vi "AttackerPenalty.vi"(4 "AI Parameters":T8={"GotoKick"={"Dist do cone a frente"=150.0, "attacker farback"=1500.0, "Perto"=300.0, "min dist to kick"=150.0, "kick eps"=0.0, "Time to transition"=0.05}, "Attacker"={"CC chute"=0.09, "CC passe"=0.045, "Kick Force"=100.0, "ball-robot Kick"=200.0, "ball-robot Pass"=0.3, "drible\nAttk"=FALSE}, "Defender"={"D max"=1700.0, "Vel p/ robô av"=1000.0, "Kick Force"=100.0, "D atk-def"=0.0, "D farback"=0.0, "drible\ndef"=FALSE, "drible\ngoalie"=FALSE}, "Timeout"={"Field/v in x"=6.0, "Dist Robots"=300, "Dist up in y"=300}, "Pose Striker"={"dist"=200.0, "Numeric"=-4.0, "dist 2"=200.0, "drible\nstriker"=FALSE}, "Dist Stop"=300.0, "D ball out"=200, "D central gap "=150.0, "T pass"=0.0, "Force ++"=0.0, "range kick"=0.0, "Chute alto"=TRUE, "Marcador novo"=TRUE, "drible"=FALSE, "D drible"=300.0, "Versão Striker"=enum."Auto", "Defesa"=enum."ManMark", "Marcador"=enum."Marcar Segundo mais perigoso", "Receptor passe"=enum."Auto", "Área"=enum."Quadrada", "Decisão\nsimples?"=FALSE} {"D drible" format="%#_13g"; "D central gap" format="%#_13g"; "Dist Stop" format="%#_13g"; "Pose Striker"."Numeric" format="%#_13g"; "Defender"."Kick Force" format="%#_13g"; "Defender"."Vel p/ robô av" format="%#_13g"; "Attacker"."ball-robot Kick" format="%#_13g"; "Attacker"."Kick Force" format="%#_13g"; "Attacker"."CC passe" format="%#_13g"; "Attacker"."CC chute" format="%#_13g"; "GotoKick"."kick eps" format="%#_13g"; "GotoKick"."min dist to kick" format="%#_13g"; "GotoKick"."Perto" format="%#_13g"; "GotoKick"."attacker farback" format="%#_13g"; "GotoKick"."Dist do cone a frente" format="%#_13g"}, 7 "IA State Input":T9={"our_robots"=[], "enemy_robots"=[], "balls"=[], "geometry"={"line_width"=0, "field_length"=0, "field_width"=0, "boundary_width"=0, "referee_width"=0, "goal_width"=0, "goal_depth"=0, "goal_wall_width"=0, "center_circle_radius"=0, "defense_radius"=0, "defense_stretch"=0, "free_kick_from_defense_dist"=0, "penalty_spot_from_field_line_dist"=0, "penalty_line_from_spot_dist"=0}, "IA Judge"={"stage"="", "command"="", "our_goalie_id"=0.0, "enemy_goalie_id"=0.0, "command enum"=enum."Halt", "Time"=enum."Azul"}, "Received Timestamp"=timestamp(0 s since 1904-01-01), "Events"={"Touch"=FALSE, "Ball out"=FALSE, "id touch"=0.0, "Ball out of \nVision"=FALSE, "Ball inside \nGoalie area"=FALSE, "Robot not responding"=FALSE, "Robots responding status"=[1.0, 1.0, 1.0, 1.0, 1.0, 1.0], "Enemy Ball \nPossession"=FALSE, "Pass State"=FALSE, "id end of pass"=0.0, "Kick"=FALSE, "Id ini Possession"=0.0, "Ball Possesion"=FALSE, "Id Possesion"=0.0, "Direct Kick"=FALSE, "2nd Strk Ativo"=FALSE}}, 8 "atacando contra?":bool=TRUE, 9 "balls":T6[](array[typedef]), 10 "geometry":T7, 11 "Robot in":T1={"id"=0, "function"=enum."Attacker", "x"=0.0, "y"=0.0, "orientation"=0.0, "v_tangent"=0.0, "v_normal"=0.0, "v_ang"=0.0, "kick_x"=0.0, "kick_z"=0.0, "dribble"=FALSE, "Timestamp"=timestamp(0 s since 1904-01-01), "estimatives"={"est_v_tangent"=0.0, "est_v_normal"=0.0, "est_vx"=0.0, "est_vy"=0.0, "Pos Robot Est"=[]}, "dest_x_kick"=0.0, "dest_y_kick"=0.0, "Gap Coord"=[], "States"=enum."GoToTangent", "Path "=[], "Path  Smooth"=[], "Dest"=[]}) -> (2 "Robot out":T1={"id"=5, "function"=enum."Attacker", "x"=-1842.5054931640625, "y"=520.60986328125, "orientation"=-2.7555055618286133, "v_tangent"=-0.08361641967936218, "v_normal"=-0.20513016702014014, "v_ang"=0.24456003022714357, "kick_x"=0.0, "kick_z"=0.0, "dribble"=FALSE, "Timestamp"=timestamp(2082758857.4639893 s since 1904-01-01), "estimatives"={"est_v_tangent"=0.0, "est_v_normal"=0.0, "est_vx"=0.0, "est_vy"=0.0, "Pos Robot Est"=[]}, "dest_x_kick"=0.0, "dest_y_kick"=0.0, "Gap Coord"=[], "States"=enum."GoToTangent", "Path "=[], "Path  Smooth"=[], "Dest"=[]})   [LabVIEW 2018]
uses:
  Core/AI Input.ctl
  Core/AI Robot.ctl
  Functions Enum.ctl
  AttackerStates.ctl
  Path Planning/RRT/PathDests.ctl
  Path Planning/RRT/PathDest.ctl
  Core/AI Ball.ctl
  Core/Field Size.ctl
  Core/AI Judge.ctl
  Command Enum.ctl
  Util/Events/Events.ctl
  AI Parameters.ctl
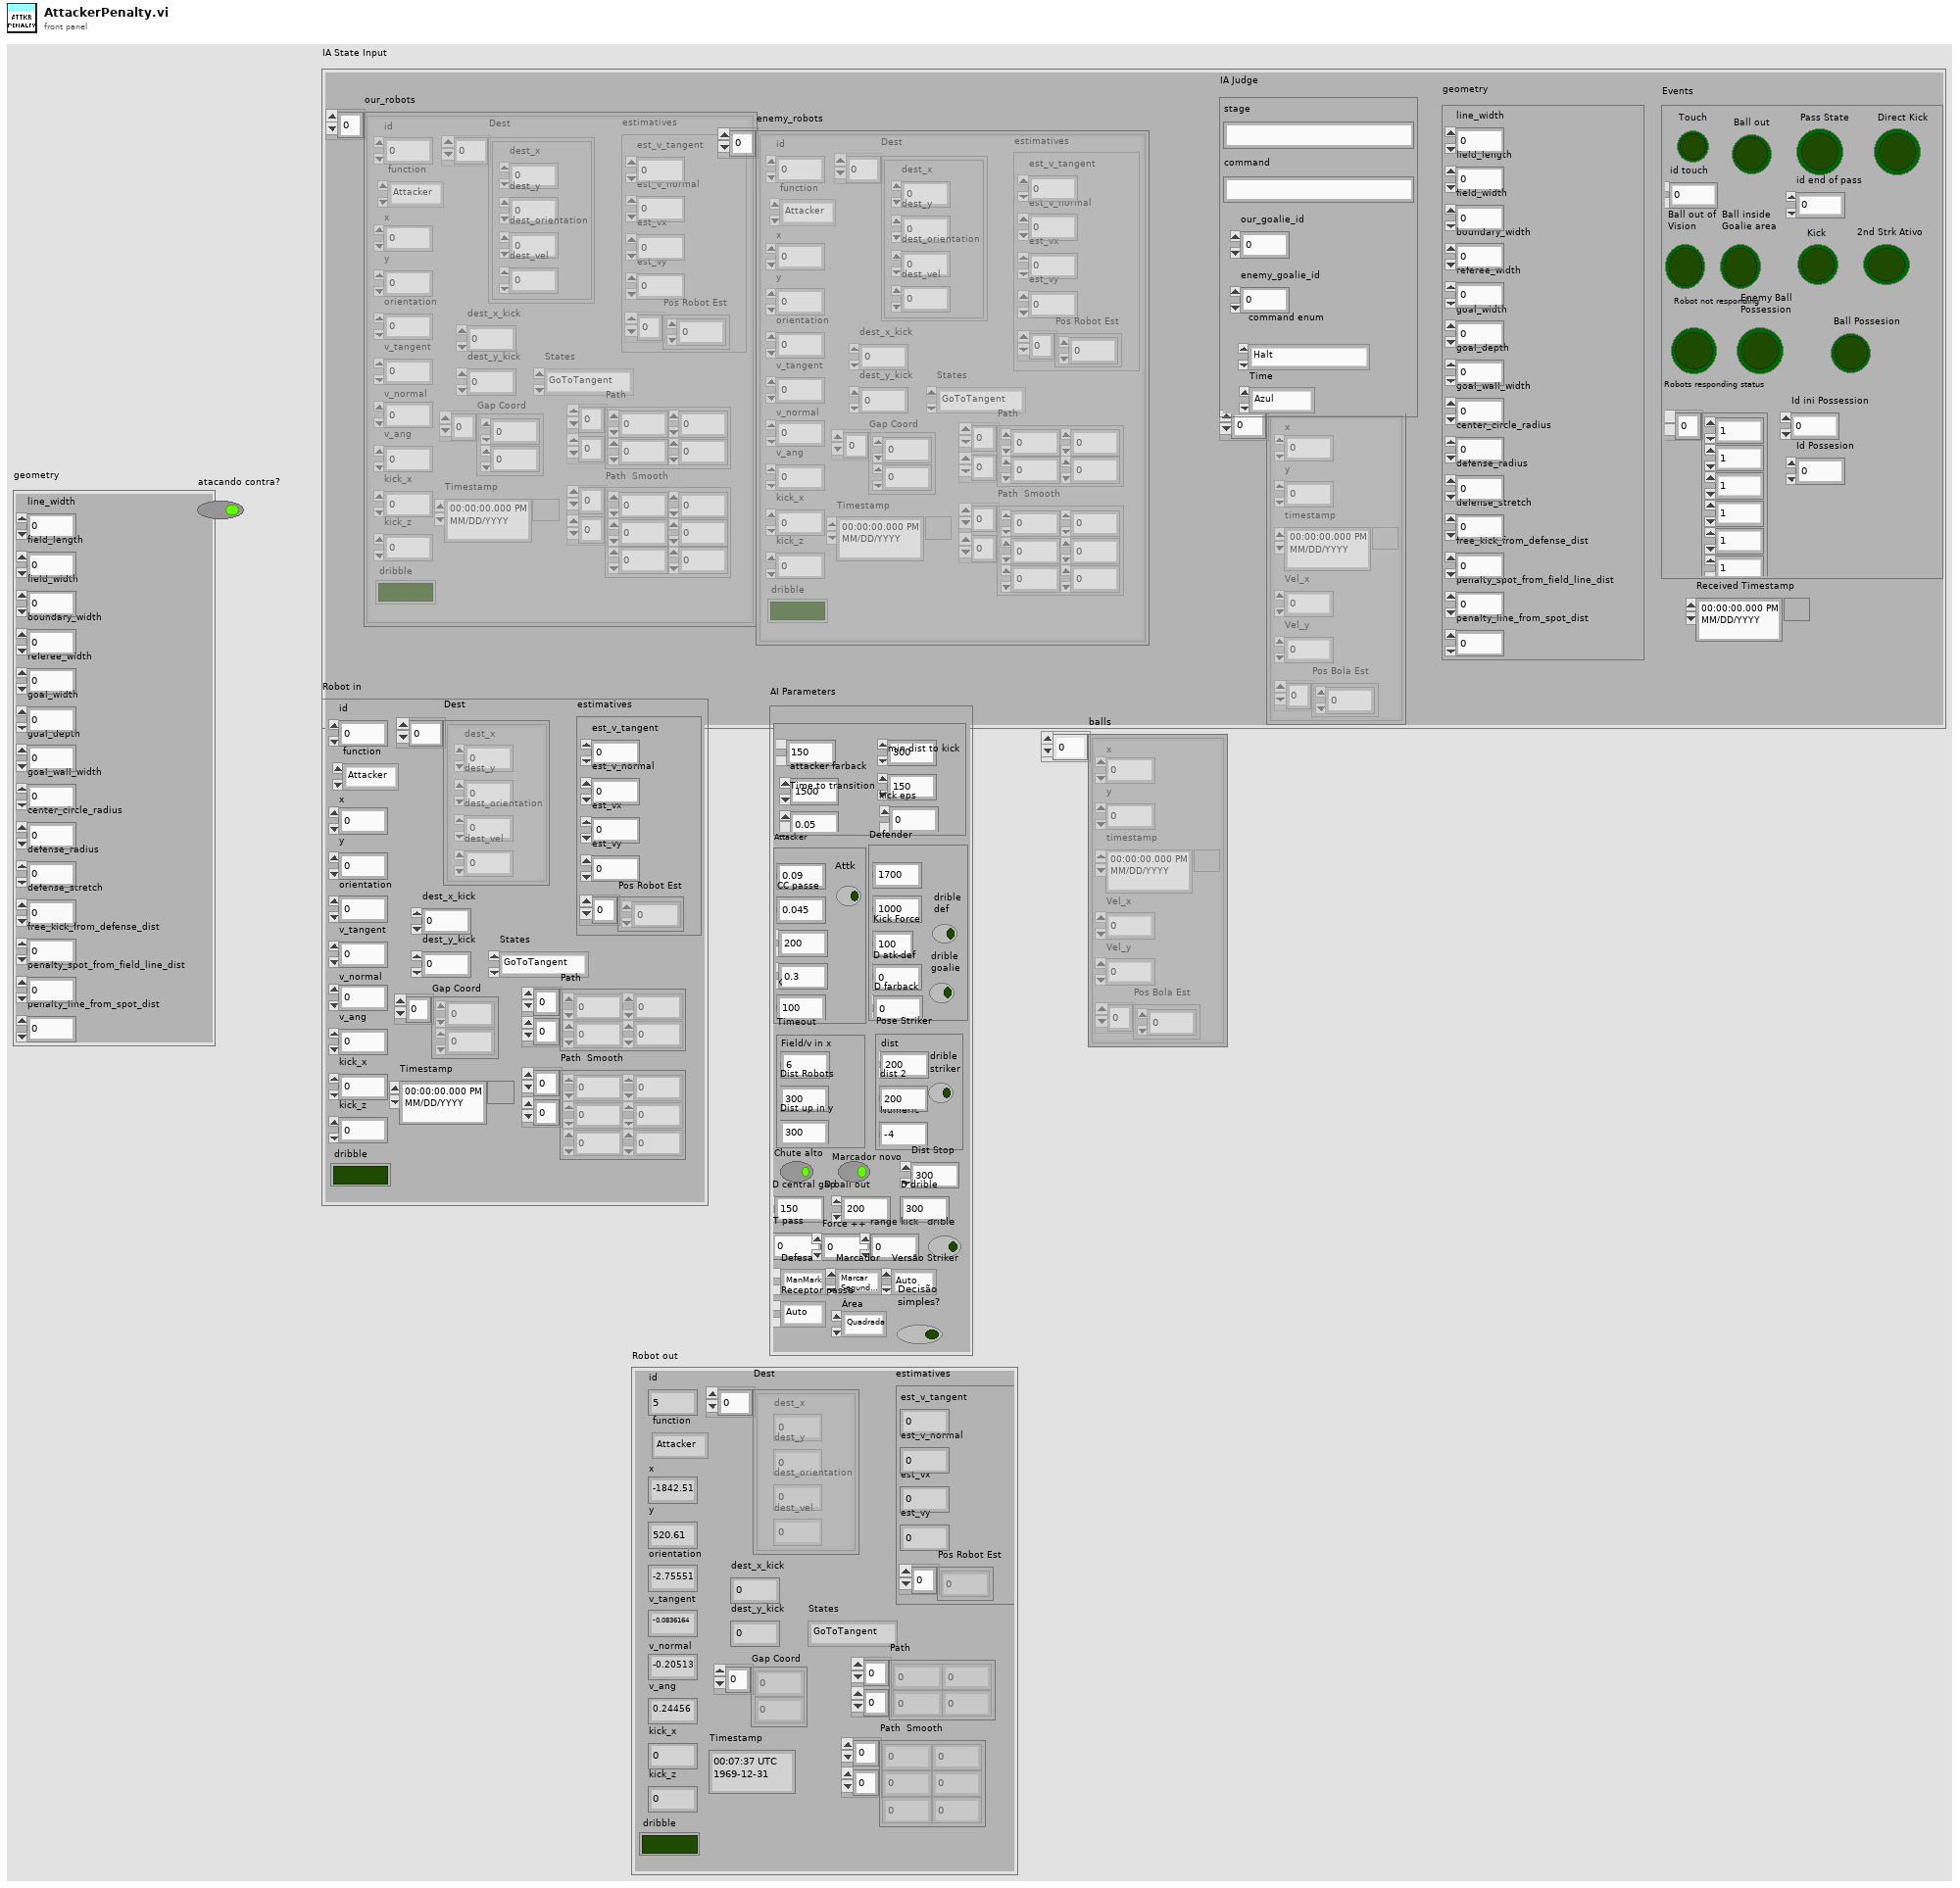
[diagram p1: front panel]
types:
  T1 = typedef "AI Robot.ctl" = cluster{"id":u32, "function":T2, "x":dbl, "y":dbl, "orientation":dbl, "v_tangent":dbl, "v_normal":dbl, "v_ang":dbl, "kick_x":dbl, "kick_z":dbl, "dribble":bool, "Timestamp":timestamp, "estimatives":cluster{"est_v_tangent":dbl, "est_v_normal":dbl, "est_vx":dbl, "est_vy":dbl, "Pos Robot Est":dbl[]}, "dest_x_kick":dbl, "dest_y_kick":dbl, "Gap Coord":dbl[], "States":T3, "Path ":dbl[][], "Path  Smooth":dbl[][], "Dest":T4}
  T2 = typedef "Functions Enum.ctl" = enum16{"2nd Striker", "Attacker", "Goalie", "Defender", "Striker", "Goto 0", "Dummy", "Kicker", "ZigZag 0", "ZigZag 1", "ZigZag 2", "ZigZag 3", "ZigZag 4", "ZigZag 5", "ZigZag 6", "ZigZag 7", "ZigZag 8", ""}
  T3 = typedef "AttackerStates.ctl" = enum16{"Pass", "GoToTangent", "BallGetting", "GoToKick", ""}
  T4 = typedef "PathDests.ctl" = T5[]
  T5 = typedef "PathDest.ctl" = cluster{"dest_x":dbl, "dest_y":dbl, "dest_orientation":dbl, "dest_vel":dbl}
  T6 = typedef "AI Ball.ctl" = cluster{"x":dbl, "y":dbl, "timestamp":timestamp, "Vel_x":dbl, "Vel_y":dbl, "Pos Bola Est":dbl[]}
  T7 = typedef "Field Size.ctl" = cluster{"line_width":u32, "field_length":u32, "field_width":u32, "boundary_width":u32, "referee_width":u32, "goal_width":u32, "goal_depth":u32, "goal_wall_width":u32, "center_circle_radius":u32, "defense_radius":u32, "defense_stretch":u32, "free_kick_from_defense_dist":u32, "penalty_spot_from_field_line_dist":u32, "penalty_line_from_spot_dist":u32}
  T8 = typedef "AI Parameters.ctl" = cluster{"GotoKick":cluster{"Dist do cone a frente":dbl, "attacker farback":dbl, "Perto":dbl, "min dist to kick":dbl, "kick eps":dbl, "Time to transition":dbl}, "Attacker":cluster{"CC chute":dbl, "CC passe":dbl, "Kick Force":dbl, "ball-robot Kick":dbl, "ball-robot Pass":dbl, "drible\nAttk":bool}, "Defender":cluster{"D max":dbl, "Vel p/ robô av":dbl, "Kick Force":dbl, "D atk-def":dbl, "D farback":dbl, "drible\ndef":bool, "drible\ngoalie":bool}, "Timeout":cluster{"Field/v in x":dbl, "Dist Robots":u32, "Dist up in y":u32}, "Pose Striker":cluster{"dist":dbl, "Numeric":dbl, "dist 2":dbl, "drible\nstriker":bool}, "Dist Stop":dbl, "D ball out":i32, "D central gap ":dbl, "T pass":dbl, "Force ++":dbl, "range kick":dbl, "Chute alto":bool, "Marcador novo":bool, "drible":bool, "D drible":dbl, "Versão Striker":enum16{"Auto", "3", "2", "1"}, "Defesa":enum16{"ManMark", "Barreira"}, "Marcador":enum16{"Marcar Segundo mais perigoso", "Marcar o mais perigoso"}, "Receptor passe":enum16{"Auto", "2nd Striker", "Striker"}, "Área":enum16{"Quadrada", "Circular"}, "Decisão\nsimples?":bool}
  T9 = typedef "AI Input.ctl" = cluster{"our_robots":T1[], "enemy_robots":T1[], "balls":T6[], "geometry":T7, "IA Judge":T10, "Received Timestamp":timestamp, "Events":T12}
  T10 = typedef "AI Judge.ctl" = cluster{"stage":string, "command":string, "our_goalie_id":dbl, "enemy_goalie_id":dbl, "command enum":T11, "Time":enum16{"Azul", "Amarelo"}}
  T11 = typedef "Command Enum.ctl" = enum16{"Halt", "Stop", "Force Start", "PKA Normal Start", "Prepare Kickoff Ally", "PKE Normal Start", "Prepare Kickoff Enemy", "Prepare Penalty Ally", "PPA Normal Start", "Prepare Penalty Enemy", "PPE Normal Start", "Direct Free Enemy", "Direct Free Ally", "Indirect Free Enemy", "Indirect Free Ally", "Timeout Enemy", "Timeout Ally", "Goal Enemy", "Goal Ally", "Ball Placement Enemy", "Ball Placement Ally", "Normal Half Time", "Extra Time Break", "Extra Half Time", "None", "Post Game"}
  T12 = typedef "Events.ctl" = cluster{"Touch":bool, "Ball out":bool, "id touch":dbl, "Ball out of \nVision":bool, "Ball inside \nGoalie area":bool, "Robot not responding":bool, "Robots responding status":dbl[], "Enemy Ball \nPossession":bool, "Pass State":bool, "id end of pass":dbl, "Kick":bool, "Id ini Possession":dbl, "Ball Possesion":bool, "Id Possesion":dbl, "Direct Kick":bool, "2nd Strk Ativo":bool}
  T13 = cluster{"CC chute":dbl, "CC passe":dbl, "Kick Force":dbl, "ball-robot Kick":dbl, "ball-robot Pass":dbl, "drible\nAttk":bool}
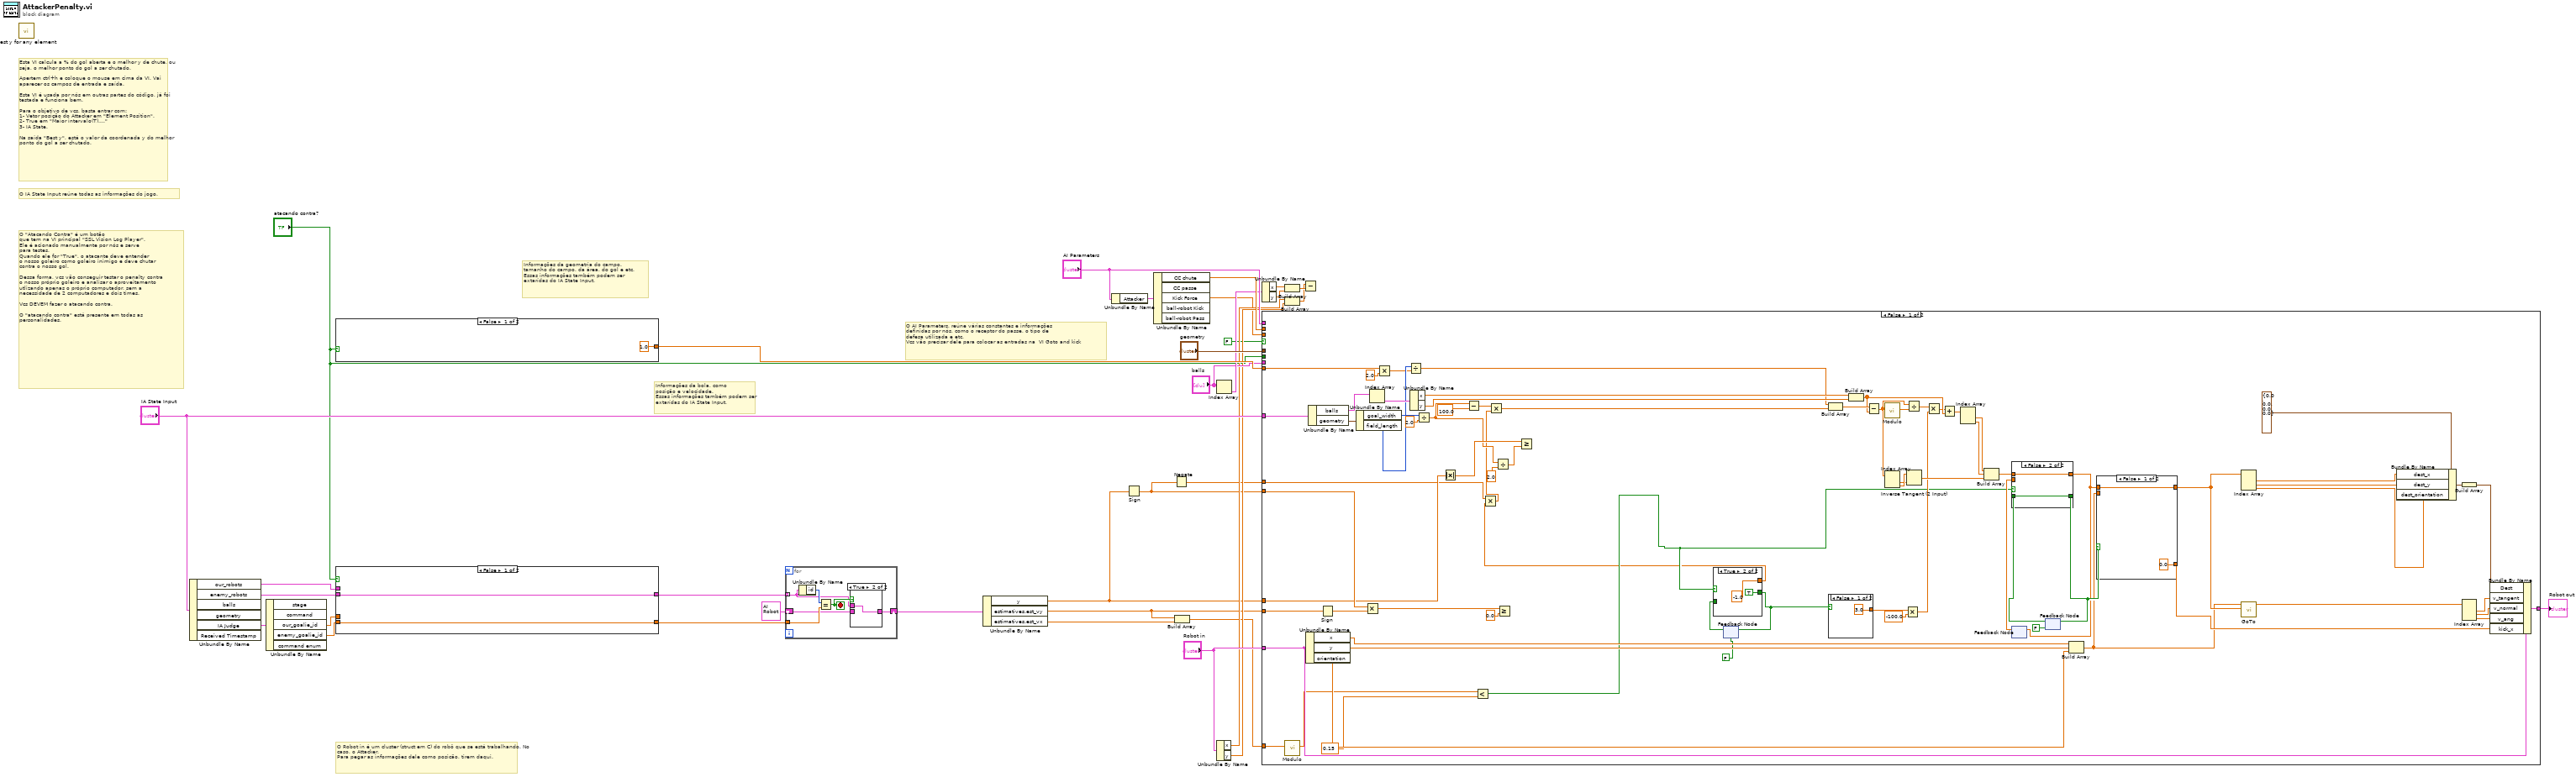
[diagram p0: block diagram]
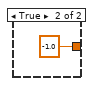
[diagram p3: hidden frame]
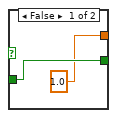
[diagram p5: hidden frame]
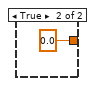
[diagram p6: hidden frame]
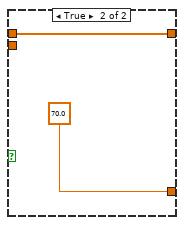
[diagram p7: hidden frame]
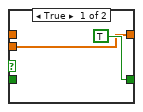
[diagram p8: hidden frame]
diagram:
  # "O \"Atacando Contra\" é um botão\nque tem na VI principal \"SSL Vision Log Player\".\nEle é acionado manualmente por nós e serve\npara testes.\nQuando ele for \"True\", o atacante deve entender \no nosso goleiro como goleiro inimigo e deve chutar\ncontra o nosso gol.\n\nDessa forma, vcs vão conseguir testar o penalty contra\no nosso próprio goleiro e analisar o aproveitamento\nutlizando apenas o próprio computador, sem a\nnecessidade de 2 computadores e dois times.\n\nVcs DEVEM fazer o atacando contra. \n\nO \"atacando contra\" está presente em todas as\npersonalidades."
  # "Informações da bola, como\nposição e velocidade.\nEssas informações também podem ser\nextarídas do IA State Input."
  # "Informações da geometria do campo.\ntamanho do campo, da área, do gol e etc.\nEssas informações também podem ser\nextarídas do IA State Input."
  # "O AI Parameters, reúne várias constantes e informações\ndefinidas por nós, como o receptor do passe, o tipo de\ndefesa utilizada e etc.\nVcs vão precisar dele para colocar as entradas na  VI Goto and kick"
  # "O Robot in é um cluster (struct em C) do robô que se está trabalhando. No caso, o Attacker.\nPara pegar as informações dele como posicão, tirem daqui."
  # "O IA State Input reúne todas as informações do jogo."
  # "Esta VI calcula a % do gol aberta e o melhor y de chute, ou seja, o melhor ponto do gol a ser chutado.\n\nApertem ctrl+h e coloque o mouse em cima da VI. Vai aparecer os campos de entrada e saída.\n\nEsta VI é usada por nós em outras partes do código, já foi testada e funciona bem.\n\nPara o objetivo de vcs, basta entrar com:\n1- Vetor posição do Attacker em \"Element Position\".\n2- True em \"Maior intervalo(T)....\"\n3- IA State.\n\nNa saída \"Best y\", está o valor da coordenada y do melhor ponto do gol a ser chutado."
  n1 = call "Best y for any element.vi"() -> ()  [unwired: 7 in, 5 out]
  n2 = Unbundle By Name("IA State Input") -> ("our_robots"=w10:T1[], "enemy_robots"=w14:T1[], "IA Judge"=w30:T10)  [unwired: 3 out]
  n3 = Unbundle By Name(w30) -> ("our_goalie_id"=w11:dbl, "enemy_goalie_id"=w12:dbl)  [unwired: 3 out]
  n4 = case shown="False" "atacando contra?" {
    tunnel: [1.0 -1.0] -> w29
    frame False {
    }
    frame True {
    }
  }
  n5 = case shown="False" "atacando contra?" {
    tunnel: [w38 w39] -> w15
    tunnel: w14 -> [w38 _]
    tunnel: [w37 w40] -> w13
    tunnel: w12 -> [w37 _]
    tunnel: w11 -> [_ w40]
    tunnel: w10 -> [_ w39]
    frame False {
    }
    frame True {
    }
  }
  n6 = for {
    tunnel: w15 -> [w42] mode=indexing
    tunnel: w13 -> [w46]
    shift-right: [w43] -> w9
    shift-left: T1 {"id"=0, "function"=enum."Attacker", "x"=0.0, "y"=0.0, "orientation"=0.0, "v_tangent"=0.0, "v_normal"=0.0, "v_ang"=0.0, "kick_x"=0.0, "kick_z"=0.0, "dribble"=FALSE, "Timestamp"=timestamp(0 s since 1904-01-01), "estimatives"={"est_v_tangent"=0.0, "est_v_normal"=0.0, "est_vx"=0.0, "est_vy"=0.0, "Pos Robot Est"=[]}, "dest_x_kick"=0.0, "dest_y_kick"=0.0, "Gap Coord"=[], "States"=enum."GoToTangent", "Path "=[], "Path  Smooth"=[], "Dest"=[]} ("Robot") -> [w41]
    stop <- w44 stop-if-true
    n7 = Unbundle By Name(w42) -> ("id"=w45:u32)
    n8 = Equal?(x=w45, y=w46) -> (x = y?=w44:bool)
    n9 = case shown="True" w44 {
      tunnel: [w47 w48] -> w43
      tunnel: w42 -> [_ w48]
      tunnel: w41 -> [w47 _]
      frame False {
      }
      frame True {
      }
    }
  }
  n10 = Unbundle By Name(w9) -> ("y"=w1:dbl, "estimatives.est_vy"=w3:dbl, "estimatives.est_vx"=w5:dbl)
  n11 = Unbundle By Name("AI Parameters") -> ("Attacker"=w34:T13)
  n12 = Sign(1:w1) -> (0:w2:dbl)
  n13 = Unbundle By Name(w34) -> ("CC chute"=w27:dbl, "Kick Force"=w8:dbl)  [unwired: 3 out]
  n14 = Negate(x=w2) -> (-x=w6:dbl)
  n15 = Build Array(w3, w5) -> (w4:dbl[])
  n16 = Index Array(array="balls") -> (element=w24:T6)  [unwired: 1 in]
  n17 = Unbundle By Name("Robot in") -> ("x"=w21:dbl, "y"=w20:dbl)
  n18 = Unbundle By Name(w24) -> ("x"=w25:dbl, "y"=w26:dbl)
  n19 = case shown="False" FALSE {
    tunnel: [w123 w138] -> w33
    tunnel: "AI Parameters" -> [_ _]
    tunnel: "IA State Input" -> [w116 _]
    tunnel: "Robot in" -> [w119 w138]
    tunnel: w29 -> [w97 _]
    tunnel: "atacando contra?" -> [_ _]
    tunnel: "geometry" -> [_ _]
    tunnel: "balls" -> [_ _]
    tunnel: w27 -> [_ _]
    tunnel: w8 -> [_ _]
    tunnel: w6 -> [w51 _]
    tunnel: w4 -> [w69 _]
    tunnel: w3 -> [w68 _]
    tunnel: w2 -> [w66 _]
    tunnel: w1 -> [w60 _]
    frame False {
      n20 = call "Modulo.vi"("2D vector"=w69) -> ("Modulo"=w62:dbl)  [unwired: 10 in]
      n21 = Unbundle By Name(w119) -> ("x"=w103:dbl, "y"=w118:dbl, "orientation"=w117:dbl)
      n22 = Unbundle By Name(w116) -> ("balls"=w102:T6[], "geometry"=w110:T7)
      n23 = Sign(1:w68) -> (0:w67:dbl)
      n24 = Unbundle By Name(w110) -> ("goal_width"=w100:u32, "field_length"=w98:u32)
      n25 = Multiply(x=w66, y=w67) -> (x*y=w65:dbl)
      n26 = Index Array(array=w102) -> (element=w115:T6)  [unwired: 1 in]
      n27 = Multiply(x=w97, y=2.0) -> (x*y=w95:dbl)
      n28 = Divide(x=w98, y=w95) -> (x/y=w92:dbl)
      n29 = Unbundle By Name(w115) -> ("x"=w114:dbl, "y"=w113:dbl)
      n30 = Divide(x=w100, y=2.0) -> (x/y=w57:dbl)
      n31 = Absolute Value(x=w60) -> (abs(x)=w59:dbl)
      n32 = Subtract(x=w57, y=100.0) -> (x-y=w93:dbl)
      n33 = Less?(x=w62, y=0.15) -> (x < y?=w52:bool)
      n34 = Divide(x=w57, y=2.0) -> (x/y=w56:dbl)
      n35 = Greater Or Equal?(x=w65, y=0.0) -> ()  [unwired: 1 out]
      n36 = Greater Or Equal?(x=w59, y=w56) -> ()  [unwired: 1 out]
      n37 = feedback #1(FALSE) -> (w54:bool)
      n38 = case shown="True" w52 {
        tunnel: [w125 TRUE] -> w55
        tunnel: w54 -> [w125 _]
        tunnel: [1.0 -1.0] -> w49
        frame False {
        }
        frame True {
        }
      }
      n39 = Multiply(x=w51, y=w49) -> (x*y=w50:dbl)
      n40 = Multiply(x=w93, y=w50) -> (x*y=w91:dbl)
      n41 = feedback-in #1(w55) -> ()
      n42 = Build Array(w92, w91) -> (w90:dbl[])
      n43 = case shown="False" w55 {
        tunnel: [3.0 0.0] -> w70
        frame False {
        }
        frame True {
        }
      }
      n44 = Build Array(w114, w113) -> (w77:dbl[])
      n45 = Subtract(x=w90, y=w77) -> (x-y=w87:dbl[])
      n46 = call "Modulo.vi"("2D vector"=w87) -> ("Modulo"=w89:dbl)  [unwired: 10 in]
      n47 = Index Array(array=w87) -> (element #1=w111:dbl, element #2=w112:dbl)  [unwired: 2 in]
      n48 = Multiply(x=w70, y=-100.0) -> (x*y=w71:dbl)
      n49 = Divide(x=w87, y=w89) -> (x/y=w88:dbl[])
      n50 = Inverse Tangent (2 Input)(1:w111, 2:w112) -> (0:w75:dbl)
      n51 = Multiply(x=w88, y=w71) -> (x*y=w76:dbl[])
      n52 = Add(x=w76, y=w77) -> (x+y=w86:dbl[])
      n53 = Index Array(array=w86) -> (element #1=w85:dbl, element #2=w84:dbl)  [unwired: 2 in]
      n54 = Build Array(w85, w84, w75) -> (w63:dbl[])
      n55 = feedback #2() -> (w73:dbl[])  [unwired: 1 in]
      n56 = feedback #3(FALSE) -> (w83:bool)
      n57 = case shown="False" w52 {
        tunnel: [TRUE w137] -> w82
        tunnel: w83 -> [_ w137]
        tunnel: w63 -> [_ w136]
        tunnel: [w134 w136] -> w74
        tunnel: w73 -> [w134 _]
        frame True {
        }
        frame False {
        }
      }
      n58 = feedback-in #2(w74) -> ()
      n59 = feedback-in #3(w82) -> ()
      n60 = Build Array(w103, w118, w117) -> (w78:dbl[])
      n61 = case shown="False" w82 {
        tunnel: [0.0 70.0] -> w80
        tunnel: w74 -> [w130 w132]
        tunnel: [w130 w132] -> w79
        tunnel: w78 -> [_ _]
        frame False {
        }
        frame True {
        }
      }
      n62 = Index Array(array=w79) -> (element #1=w108:dbl, element #2=w107:dbl, element #3=w106:dbl)  [unwired: 3 in]
      n63 = call "GoTo.vi"("Target"=w79, "Position"=w78) -> ("Output\nVelocity"=w122:dbl[])  [unwired: 8 in, 1 out]
      n64 = Bundle By Name(cluster=T5 {"dest_x"=0.0, "dest_y"=0.0, "dest_orientation"=0.0, "dest_vel"=0.0} ("element"), "dest_x"=w108, "dest_y"=w107, "dest_orientation"=w106) -> (w105:T5)
      n65 = Build Array(w105) -> (w104:T5[])
      n66 = Index Array(array=w122) -> (element #1=w121:dbl, element #2=w120:dbl, element #3=w101:dbl)  [unwired: 3 in]
      n67 = Bundle By Name(cluster=w119, "Dest"=w104, "v_tangent"=w121, "v_normal"=w120, "v_ang"=w101, "kick_x"=w80) -> (w123:T1)
    }
    frame True {
    }
  }
  "Robot out" <- w33
  n68 = Build Array(w25, w26) -> (w19:dbl[])
  n69 = Build Array(w21, w20) -> (w18:dbl[])
  n70 = Subtract(x=w18, y=w19) -> ()  [unwired: 1 out]
